vi "FAM Initialization.vi"(8 "error in (no error)":errorcluster, 11 "Cluster":T1={"FPGA"={"Target"=enum."4", "Channel"=enum."4", "Ref1"=refnum, "Ref2"=refnum}, "10MHzRef"=FALSE, "FamInit"=0}) -> (0 "error out":errorcluster, 2 "FAM Initialized?":bool)   [LabVIEW 2018]
uses:
  Controls/HWCluster.ctl
  Controls/Clusts/FPGA_Config_Clust.ctl
  Controls/Enums/TargetNumber.ctl
  <vilib>/Utility/error.llb/Error Cluster From Error Code.vi
  <vilib>/rvi/errors/niLvFpgaAdjustHostInterfaceError.vi
  <vilib>/rvi/interface/nirviReadWriteControl/nirviReadWriteControl.xnode
  NiFpgaLv.dll
  <vilib>/rvi/interface/Simulation/niFpgaSimulationCallBeginRW.vi
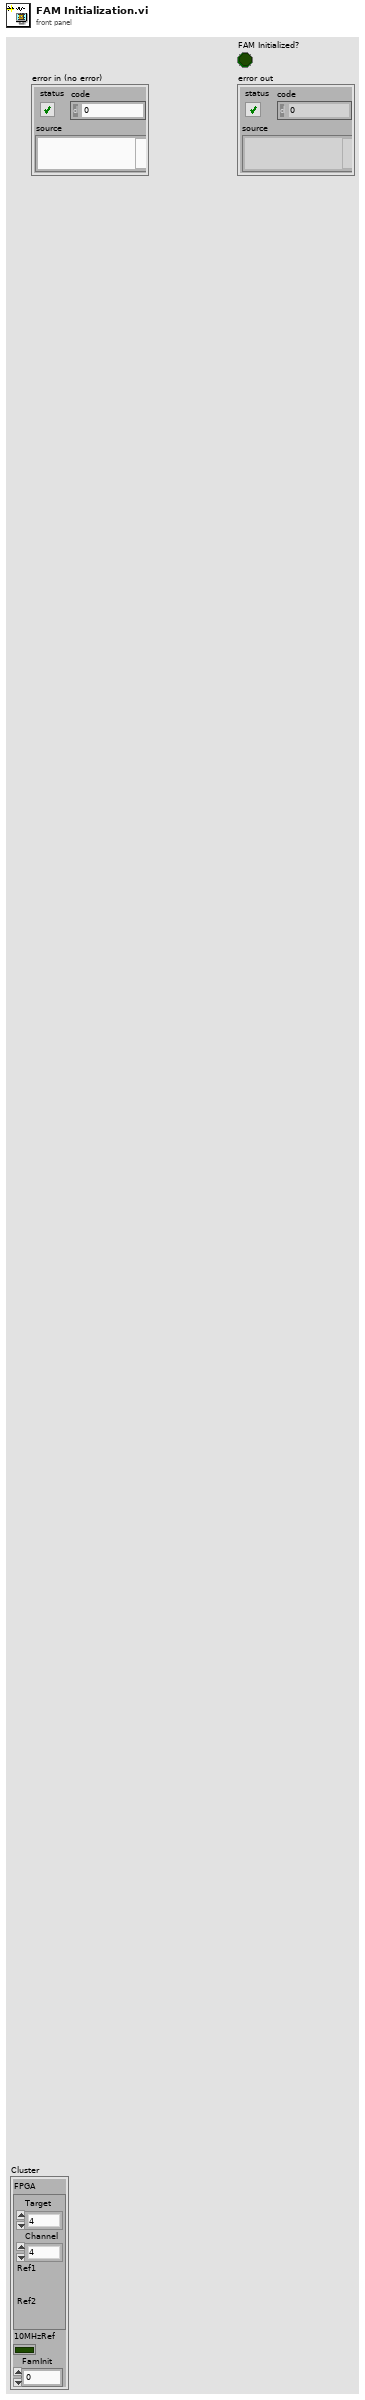
[diagram p1: front panel]
types:
  T1 = typedef "HWCluster.ctl" = cluster{"FPGA":T2, "10MHzRef":bool, "FamInit":i32}
  T2 = typedef "FPGA_Config_Clust.ctl" = cluster{"Target":T3, "Channel":T3, "Ref1":refnum<k20>, "Ref2":refnum<k20>}
  T3 = typedef "TargetNumber.ctl" = enum16{"1", "2", "3", "4"}
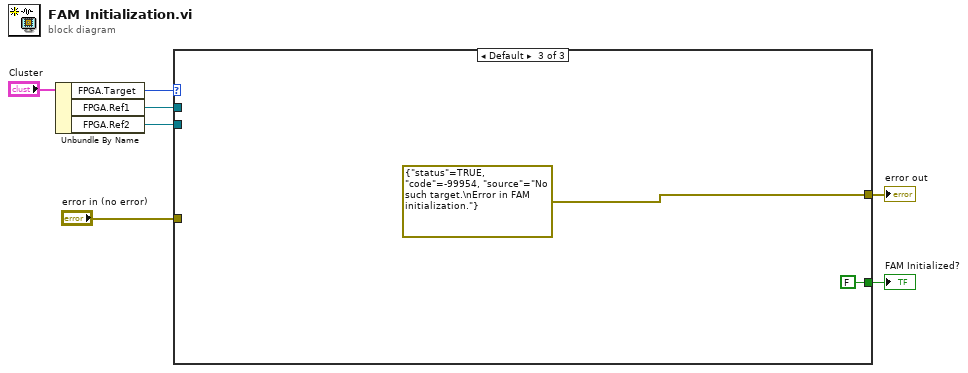
[diagram p0: block diagram]
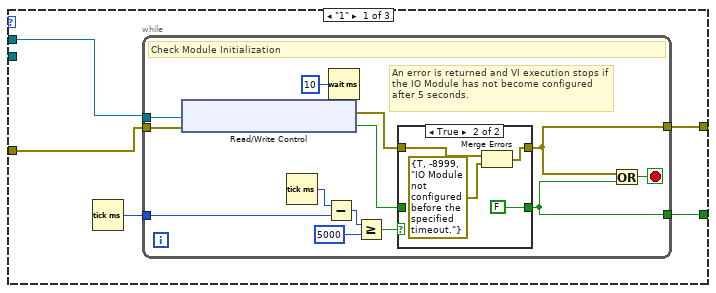
[diagram p2: hidden frame]
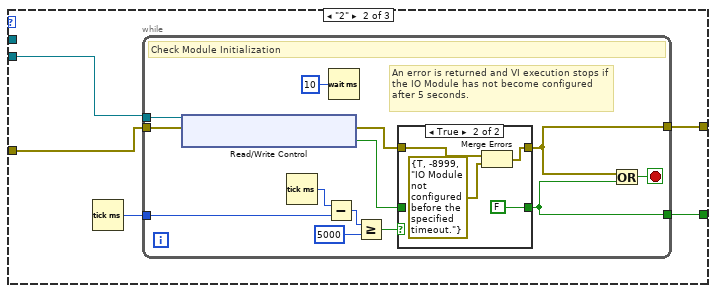
[diagram p4: hidden frame]
diagram:
  n1 = Unbundle By Name("Cluster") -> ("FPGA.Target"=w4:T3, "FPGA.Ref1"=w3:refnum<k20>, "FPGA.Ref2"=w2:refnum<k20>)
  n2 = case shown="Default" w4 {
    tunnel: [w11 w35 errorcluster {"status"=TRUE, "code"=-99954, "source"="No such target.\nError in FAM initialization."} ("error IO")] -> w7
    tunnel: [w10 w34 FALSE ("Configured?")] -> w6
    tunnel: w3 -> [w9 _ _]
    tunnel: w2 -> [_ w33 _]
    tunnel: "error in (no error)" -> [w8 w32 _]
    frame "1" {
      n3 = Tick Count (ms)() -> (millisecond timer value=w12:u32)
      n4 = while {
        tunnel: [w13] -> w11
        tunnel: w9 -> [w17]
        tunnel: w8 -> [w16]
        tunnel: w12 -> [w15]
        tunnel: [w14] -> w10
        stop <- w22 stop-if-true
        # "An error is returned and VI execution stops if the IO Module has not become configured after 5 seconds."
        # "Check Module Initialization"
        n5 = xnode "Read/Write Control"("FPGA VI Reference In"=w17, "error in"=w16) -> ("error out"=w20:errorcluster, "IO Module\\Initialization Done"=w21:bool)  [unwired: 1 out]
        n6 = Tick Count (ms)() -> (millisecond timer value=w19:u32)
        n7 = Subtract(x=w19, y=w15) -> (x-y=w18:u32)
        n8 = Wait (ms)(milliseconds to wait=u32 10) -> ()  [unwired: 1 out]
        n9 = Greater Or Equal?(x=w18, y=u32 5000) -> (x >= y?=w23:bool)
        n10 = case shown="True" w23 {
          tunnel: [w26 FALSE ("Configured?")] -> w14
          tunnel: w21 -> [w26 _]
          tunnel: [w27 w30] -> w13
          tunnel: w20 -> [w27 w28]
          frame False {
          }
          frame True {
            n11 = Merge Errors(w28, errorcluster {"status"=TRUE, "code"=-8999, "source"="IO Module not configured before the specified timeout."} ("error in")) -> (w30:errorcluster)
          }
        }
        n12 = Or(x=w13, y=w14) -> (x .or. y?=w22:bool)
      }
    }
    frame "2" {
      n13 = Tick Count (ms)() -> (millisecond timer value=w36:u32)
      n14 = while {
        tunnel: [w37] -> w35
        tunnel: w33 -> [w41]
        tunnel: w32 -> [w40]
        tunnel: w36 -> [w39]
        tunnel: [w38] -> w34
        stop <- w46 stop-if-true
        # "An error is returned and VI execution stops if the IO Module has not become configured after 5 seconds."
        # "Check Module Initialization"
        n15 = xnode "Read/Write Control"("FPGA VI Reference In"=w41, "error in"=w40) -> ("error out"=w44:errorcluster, "IO Module\\Initialization Done"=w45:bool)  [unwired: 1 out]
        n16 = Tick Count (ms)() -> (millisecond timer value=w43:u32)
        n17 = Subtract(x=w43, y=w39) -> (x-y=w42:u32)
        n18 = Wait (ms)(milliseconds to wait=u32 10) -> ()  [unwired: 1 out]
        n19 = Greater Or Equal?(x=w42, y=u32 5000) -> (x >= y?=w47:bool)
        n20 = case shown="True" w47 {
          tunnel: [w50 FALSE ("Configured?")] -> w38
          tunnel: w45 -> [w50 _]
          tunnel: [w51 w54] -> w37
          tunnel: w44 -> [w51 w52]
          frame False {
          }
          frame True {
            n21 = Merge Errors(w52, errorcluster {"status"=TRUE, "code"=-8999, "source"="IO Module not configured before the specified timeout."} ("error in")) -> (w54:errorcluster)
          }
        }
        n22 = Or(x=w37, y=w38) -> (x .or. y?=w46:bool)
      }
    }
    frame Default {
    }
  }
  "error out" <- w7
  "FAM Initialized?" <- w6
